vi "Double Mouse Test.vi"() -> ()   [LabVIEW 2011]
uses:
  <vilib>/vision/NI_Vision_Development_Module.lvlib
panel:
  out "Crop":T1(plugin-control)
  out "x < y?":bool
  in  "Threshold":dbl(slide)=51.515151515151516 scale=0.0..60.0
  in  "Standard Deviation":dbl=3.0
  in  "Kernel Size":i32=11
  out "Image":T1(plugin-control)
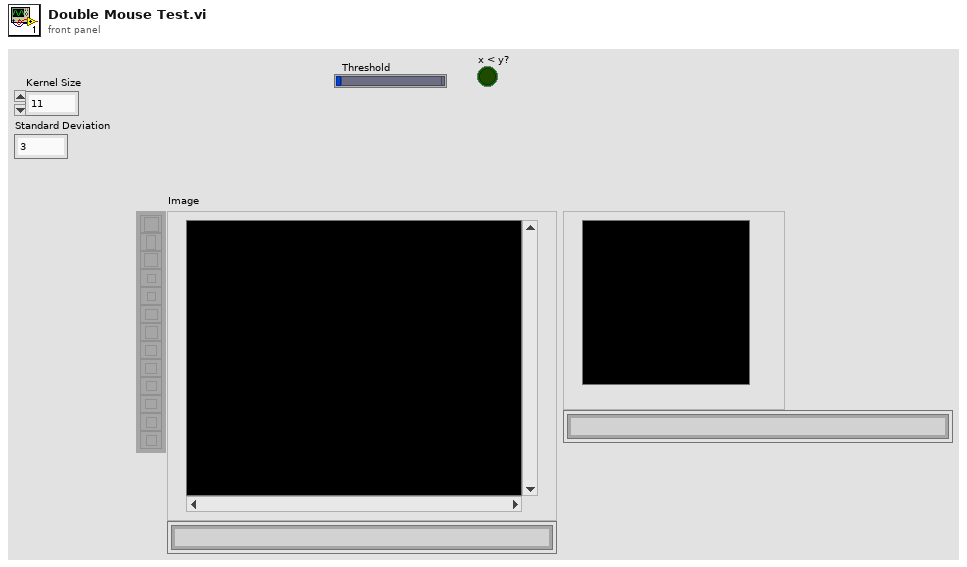
[diagram p1: front panel]
types:
  T1 = typedef "IMAQ Image.ctl" = refnum<image>
  T2 = typedef "Image Type" = u32
  T3 = cluster{"Width":i32, "Height":i32, "N Gaussians":i32}
  T4 = cluster{"Area":dbl, "Number of Holes":dbl, "Bounding Rect":cluster{"Left":dbl, "Top":dbl, "Right":dbl, "Bottom":dbl}, "Center of Mass":cluster{"X":dbl, "Y":dbl}, "Orientation":dbl, "Dimensions":cluster{"Width":dbl, "Height":dbl}}[]
  T5 = cluster{"Particle 2 Index":i32, "Particle 1 Index":i32, "Distance":dbl}[]
  T6 = cluster{"Particle 2 Index":i32, "Particle 1 Index":i32, "Distance":dbl}
  T7 = cluster{"Area":dbl, "Number of Holes":dbl, "Bounding Rect":cluster{"Left":dbl, "Top":dbl, "Right":dbl, "Bottom":dbl}, "Center of Mass":cluster{"X":dbl, "Y":dbl}, "Orientation":dbl, "Dimensions":cluster{"Width":dbl, "Height":dbl}}
  T8 = cluster{"Left":dbl, "Top":dbl, "Right":dbl, "Bottom":dbl}
  T9 = cluster{"Left":dbl, "Top":dbl, "Right":dbl, "Bottom":dbl}[]
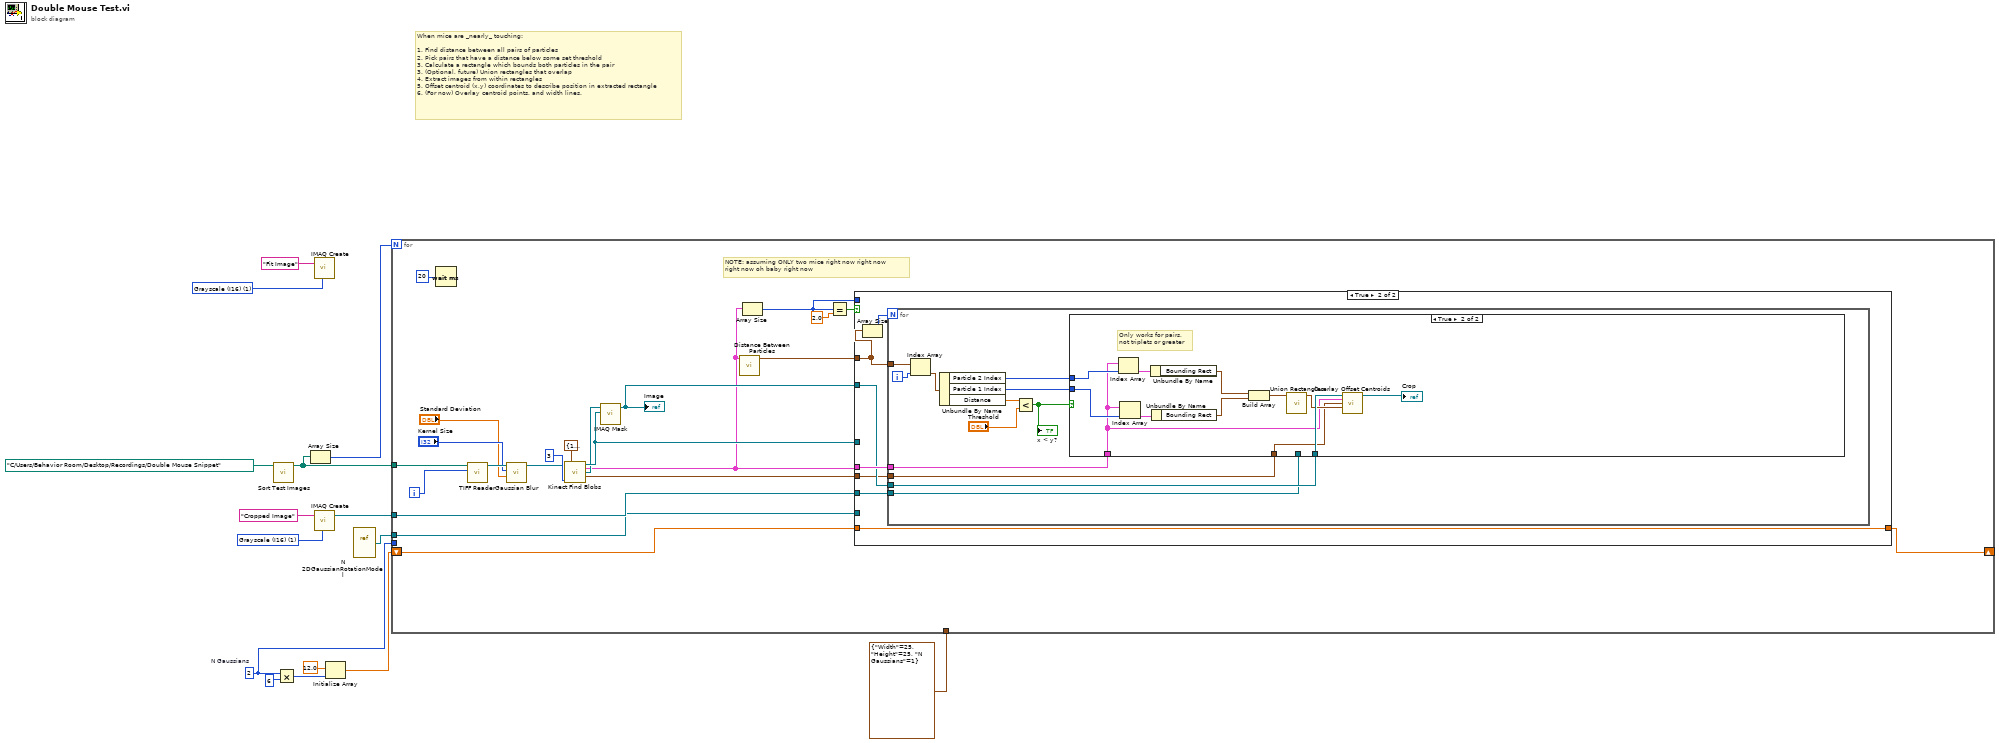
[diagram p0: block diagram]
diagram:
  w2 = T2 1 items=["Grayscale (U8)", "Grayscale (I16)", "Grayscale (SGL)", "Complex (CSG)", "RGB (U32)", "HSL (U32)", "RGB (U64)", "Grayscale (U16)"] ("Image Type")
  w4 = 2  # N Gaussians
  w12 = T2 1 items=["Grayscale (U8)", "Grayscale (I16)", "Grayscale (SGL)", "Complex (CSG)", "RGB (U32)", "HSL (U32)", "RGB (U64)", "Grayscale (U16)"] ("Image Type")
  # "When mice are _nearly_ touching:\n\n1. Find distance between all pairs of particles\n2. Pick pairs that have a distance below some set threshold\n3. Calculate a rectangle which bounds both particles in the pair\n3. (Optional, future) Union rectangles that overlap\n4. Extract images from within rectangles\n5. Offset centroid (x,y) coordinates to describe position in extracted rectangle\n6. (For now) Overlay centroid points, and width lines."
  n1 = call "Sort Test Images.vi"("path"=path "C:/Users/Behavior Room/Desktop/Recordings/Double Mouse Snippet") -> ("Array"=w14:path[])  [unwired: 10 in]
  n2 = Multiply(x=w4, y=6 ("dimension size")) -> (x*y=w7:i32)
  n3 = Array Size(array=w14) -> (size(s)=w15:i32)
  n4 = call "IMAQ Create"("Image Name"="Fit Image", "Image Type"=w2) -> ()  [unwired: 3 in, 2 out]
  n5 = call "IMAQ Create"("Image Name"="Cropped Image", "Image Type"=w12) -> ("New Image"=w11:T1)  [unwired: 3 in, 1 out]
  n6 = Initialize Array(12.0 ("element"), w7) -> (w3:dbl[])
  n7 = vi-ref "N 2DGaussianRotationModel.vi"() -> (w9:refnum<vi>)
  n8 = for {
    N: w15 -> [_]
    tunnel: w14 -> [w37]
    tunnel: w11 -> [w33]
    tunnel: w4 -> [_]
    tunnel: w9 -> [w31]
    tunnel: T3 {"Width"=25, "Height"=25, "N Gaussians"=1} -> [_]
    shift-right: [w29] -> _
    shift-left: w3 -> [w30]
    i -> [w36]
    # "NOTE: assuming ONLY two mice right now right now\nright now oh baby right now"
    n9 = Wait (ms)(milliseconds to wait=u32 20) -> ()  [unwired: 1 out]
    n10 = call "TIFF Reader.vi"("index"=w36, "Array"=w37) -> ("Image Out"=w27:T1)  [unwired: 9 in]
    n11 = call "Gaussian Blur.vi"("Standard Deviation"="Standard Deviation", "Kernel Size"="Kernel Size", "Image"=w27) -> ("Image Out"=w24:T1)  [unwired: 8 in]
    n12 = call "Kinect Find Blobs.vi"("Image Src"=w24, "Range"=cluster{"Lower value":sgl, "Upper value":sgl} {"Lower value"=100.0, "Upper value"=32768.0}, "Number of Erosion"=3) -> ("Masked Image Out"=w28:T1, "Particle Reports (Pixels)"=w21:T4, "Src Image Out"=w23:T1, "Ellipse Data"=w16:cluster{"Major":dbl, "Minor":dbl}[])  [unwired: 9 in]
    n13 = call "IMAQ Mask"("Image Mask"=w28, "Image Src"=w23) -> ("Image Dst Out"=w22:T1)  [unwired: 3 in, 1 out]
    "Image" <- w22
    n14 = call "Distance Between Particles.vi"("Particle Reports"=w21) -> ("output array"=w18:T5)  [unwired: 10 in]
    n15 = Array Size(array=w21) -> (size(s)=w17:i32)
    n16 = Equal?(x=w17, y=2.0) -> (x = y?=w20:bool)
    n17 = case shown="True" w20 {
      tunnel: w21 -> [_ w42]
      tunnel: w33 -> [_ w40]
      tunnel: w31 -> [_ _]
      tunnel: [w38 w45] -> w29
      tunnel: w30 -> [w38 w45]
      tunnel: w28 -> [_ _]
      tunnel: w22 -> [_ w41]
      tunnel: w18 -> [_ w43]
      tunnel: w17 -> [_ _]
      tunnel: w16 -> [_ w39]
      frame False {
      }
      frame True {
        n18 = Array Size(array=w43) -> (size(s)=w44:i32)
        n19 = for {
          N: w44 -> [_]
          tunnel: w43 -> [w55]
          tunnel: w42 -> [w52]
          tunnel: w41 -> [w49]
          tunnel: w40 -> [w47]
          tunnel: w39 -> [w46]
          i -> [w54]
          n20 = Index Array(array=w55, index=w54) -> (element=w53:T6)
          n21 = Unbundle By Name(w53) -> ("Particle 2 Index"=w51:i32, "Particle 1 Index"=w50:i32, "Distance"=w57:dbl)
          n22 = Less?(x=w57, y="Threshold") -> (x < y?=w48:bool)
          "x < y?" <- w48
          n23 = case shown="True" w48 {
            tunnel: w52 -> [_ w60]
            tunnel: w51 -> [_ w69]
            tunnel: w50 -> [_ w68]
            tunnel: w49 -> [_ w62]
            tunnel: w47 -> [_ _]
            tunnel: w46 -> [_ w58]
            frame False {
            }
            frame True {
              # "Only works for pairs, \nnot triplets or greater"
              n24 = Index Array(array=w60, index=w69) -> (element=w66:T7)
              n25 = Index Array(array=w60, index=w68) -> (element=w67:T7)
              n26 = Unbundle By Name(w66) -> ("Bounding Rect"=w65:T8)
              n27 = Unbundle By Name(w67) -> ("Bounding Rect"=w64:T8)
              n28 = Build Array(w65, w64) -> (w63:T9)
              n29 = call "Union Rectangles.vi"("Rectangles"=w63) -> ("Bounding Rect"=w61:T8)  [unwired: 10 in]
              n30 = call "Overlay Offset Centroids.vi"("Image"=w62, "Particle Reports (Pixels)"=w60, "Ellipse Data"=w58, "Bounding Rect"=w61) -> ("Image Out"=→"Crop":T1)  [unwired: 11 in]
            }
          }
        }
      }
    }
  }
